vi "GLOBAL on RT.vi"() -> ()   [LabVIEW 2015]
panel:
  in  "STOP Remote (UART)":bool
  in  "STOP DRIVE":bool
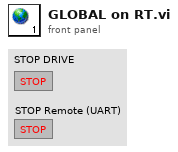
[diagram p1: front panel]
diagram:
